vi "Actor Core.vi"(8 "error in":errorcluster, 11 "IViewModel In":refnum<class "IViewModel.lvclass">) -> (0 "error out":errorcluster, 3 "Actor out":refnum<class "Actor.lvclass">)   [LabVIEW 2015, in "IViewModel.lvlib" / "IViewModel.lvclass"]
doc: "(<B>Filename</B>: Actor Framework.lvlib:Actor.lvclass:Actor Core.vi)\n\nReceives messages to the actor, reacts to them, and initiates any error handling that may shut the actor down.\n\nDescendant classes may override this VI to append parallel tasks for the actor to complete while it handles messages. Overrides use the Call Parent Method node."
uses:
  IViewModel.lvclass
  <vilib>/ActorFramework/Actor/Actor.lvclass
  <vilib>/ActorFramework/Actor/Actor.lvclass/Actor.ctl
  <vilib>/ActorFramework/Message Enqueuer/Message Enqueuer.lvclass/Message Enqueuer.ctl
  <vilib>/ActorFramework/Message Enqueuer/Init from Existing Queue.vi
  <vilib>/ActorFramework/Message Enqueuer/Message Enqueuer.lvclass
  IViewManager/IViewManager/IViewManager.lvclass
  AutoRegistration/ActorAutoRegistration/ActorAutoRegistration.lvclass
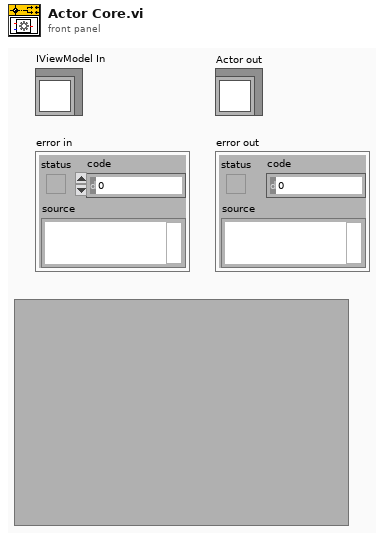
[diagram p1: front panel]
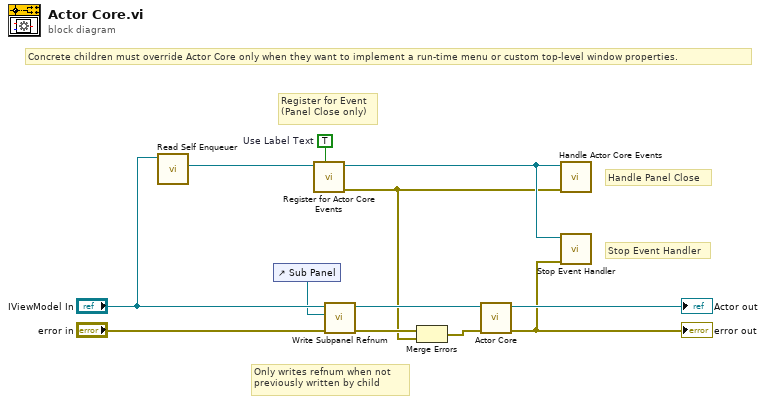
[diagram p0: block diagram]
diagram:
  w6 = TRUE  # Use Label Text
  # "Register for Event\n(Panel Close only)"
  # "Stop Event Handler"
  # "Handle Panel Close"
  # "Only writes refnum when not\npreviously written by child"
  # "Concrete children must override Actor Core only when they want to implement a run-time menu or custom top-level window properties."
  n1 = call <vilib>:"Read Self Enqueuer.vi"("Actor"="IViewModel In") -> ("Self Enqueuer"=w4:refnum<class "Message Enqueuer.lvclass">)  [unwired: 10 in]
  n2 = control-ref of="Sub Panel"() -> (w1:refnum<vi>)
  n3 = call "Register for Actor Core Events.vi"("Use Label Text (F=Use Caption)"=w6, "Actor Enqueuer"=w4) -> ("error out"=w7:errorcluster, "ActorAutoRegistration Out"=w10:refnum<class "ActorAutoRegistration.lvclass">)  [unwired: 8 in]
  n4 = call "Write Subpanel Refnum.vi"("error in (no error)"="error in", "SubPnl Refnum"=w1, "IViewModel In"="IViewModel In") -> ("error out"=w9:errorcluster, "IViewModel Out"=w11:refnum<class "IViewModel.lvclass">)  [unwired: 7 in]
  n5 = Merge Errors(w9, w7) -> (w8:errorcluster)
  n6 = call-parent "Actor Core.vi"("error in"=w8, "IViewable In"=w11) -> ("error out"=w3:errorcluster, "Actor out"=→"Actor out":refnum<class "Actor.lvclass">)  [unwired: 8 in]
  "error out" <- w3
  n7 = call-dynamic "Handle Actor Core Events.vi"("error in (no error)"=w7, "ActorAutoRegistration in"=w10) -> ()  [unwired: 9 in, 1 out]
  n8 = call-dynamic "Stop Event Handler.vi"("error in (no error)"=w3, "ActorAutoRegistration in"=w10) -> ()  [unwired: 9 in, 1 out]
